vi "Queue Ball Element cam2.vi"(8 "error in (no error)":errorcluster, 11 "Image in":T1) -> (0 "error out":errorcluster)   [LabVIEW 2023]
uses:
  <vilib>/vision/Image Controls.llb/IMAQ Image.ctl
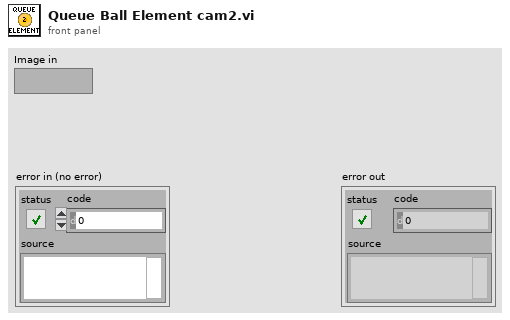
[diagram p1: front panel]
types:
  T1 = typedef "IMAQ Image.ctl" = refnum<image>
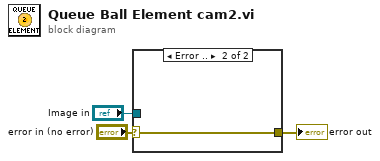
[diagram p0: block diagram]
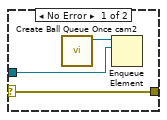
[diagram p2: hidden frame]
diagram:
  n1 = case shown="Error .." "error in (no error)" {
    selector: "error in (no error)" -> [w5 w7]
    tunnel: [w5 w7] -> w2
    tunnel: "Image in" -> [w4 _]
    frame No Error {
      n2 = call "Create Ball Queue Once cam2.vi"() -> ("queue out"=w6:refnum<queue>)  [unwired: 11 in]
      n3 = Enqueue Element(queue=w6, element=w4) -> ()  [unwired: 2 in, 3 out]
    }
    frame Error {
    }
  }
  "error out" <- w2
